vi "CRYSet Splitter Vertical Horizon Info.vi"(10 "DataView Idx":i32, 11 "spliter array":refnum<vi>[](array[refnum])) -> ()   [LabVIEW 2013]
uses:
  CRYNew View Global.vi
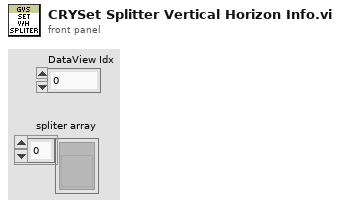
[diagram p1: front panel]
types:
  T1 = typedef "Graph Main Info Cluster.ctl" = cluster{"Selected_BarIdx":i32, "Selected_PanelIdx":i32, "Graph Main VIRef":refnum<vi>, "ToolBarClick":bool, "Spliter Ref Array":refnum<vi>[], "Panel Ref Array":refnum<vi>[], "Spliter_matrix":i32[][], "Panel_matrix":i32[][], "child_spliterIdx_matrix":i32[][], "split_pos_matrix":i32[][], "Title State":bool, "sQueueName":string, "Frame nID":i32, "Graph VIRef Array":cluster{"Graph VIRef":refnum<vi>, "Panel Idx":i32, "Frame VIRef":refnum<vi>, "Icon Ring":i32, "Graph Type":string}[], "View Type":string}
  T2 = typedef "SpliterBar.ctl" = cluster{"HBar":bool, "IsVertical":bool}
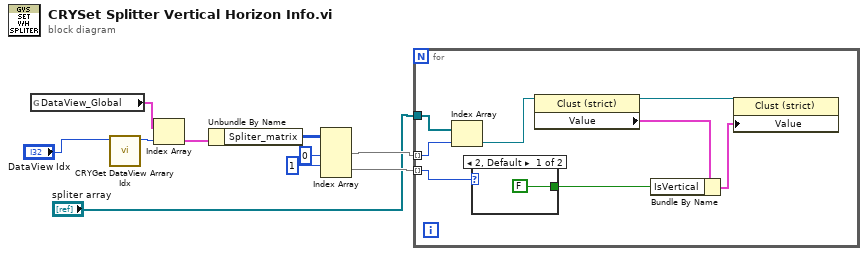
[diagram p0: block diagram]
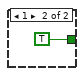
[diagram p2: hidden frame]
diagram:
  n1 = global read "CRYNew View Global.vi" "DataView_Global"() -> (w9:T1[])
  n2 = call "CRYGet DataView Arrary Idx.vi"("DataView Idx In"="DataView Idx") -> ("DataView Arrary Idx out"=w8:i32)  [unwired: 10 in]
  n3 = Index Array(array=w9, index=w8) -> (element=w7:T1)
  n4 = Unbundle By Name(w7) -> ("Spliter_matrix"=w6:i32[][])
  n5 = Index Array(array=w6, index (row) #1=0 ("index (row)"), index (row) #2=1 ("index (row)")) -> (element #1=w3:i32[], element #2=w2:i32[])  [unwired: 2 in]
  n6 = for {
    tunnel: w3 -> [w17] mode=indexing
    tunnel: w2 -> [w12] mode=indexing
    tunnel: "spliter array" -> [w18]
    n7 = Index Array(array=w18, index=w17) -> (element=w16:refnum<vi>)
    n8 = case shown="2, Default" w12 {
      tunnel: [FALSE TRUE] -> w11
      frame 2, Default {
      }
      frame 1 {
      }
    }
    n9 = property class="Clust (strict)"(reference=w16) -> (reference out=w14:refnum<vi>, "Value"=w15:T2)  [unwired: 1 in, 1 out]
    n10 = Bundle By Name(cluster=w15, "IsVertical"=w11) -> (w13:T2)
    n11 = property class="Clust (strict)"(reference=w14, "Value"=w13) -> ()  [unwired: 1 in, 2 out]
  }
